vi "Device Level, Process Single Pulse.vi"(5 "filepath":path, 6 "Waveform Filtered Zoom":bool=TRUE, 7 "Waveform Zoom":bool, 8 "error in":errorcluster, 9 "Average Size":dbl=15.0, 10 "Resistance (ohms)":dbl=500.0 format="%.1f", 11 "waveform array":waveform(dbl)={"t0"=timestamp(3474563448.844 s since 1904-01-01), "dt"=4e-06, "Y"=[]}) -> (0 "error out":errorcluster, 1 "Input Parameters":T1[](array[typedef]) {"Value" format="%#.3f"}, 2 "Results":T1[](array[typedef]) {"Value" format="%#.3f"}, 3 "waveform filtered":waveform(dbl)(graph)={"t0"=timestamp(3472747248.0780005 s since 1904-01-01), "dt"=2e-06, "Y"=[]})   [LabVIEW 2010]
doc: "This function processes a single pulse waveform."
uses:
  Generic/Waveform Attribute/Waveform Attribute Cluster.ctl
panel:
  out "waveform":waveform(dbl)(graph)={"t0"=timestamp(3473168095.069 s since 1904-01-01), "dt"=2e-06, "Y"=[]}
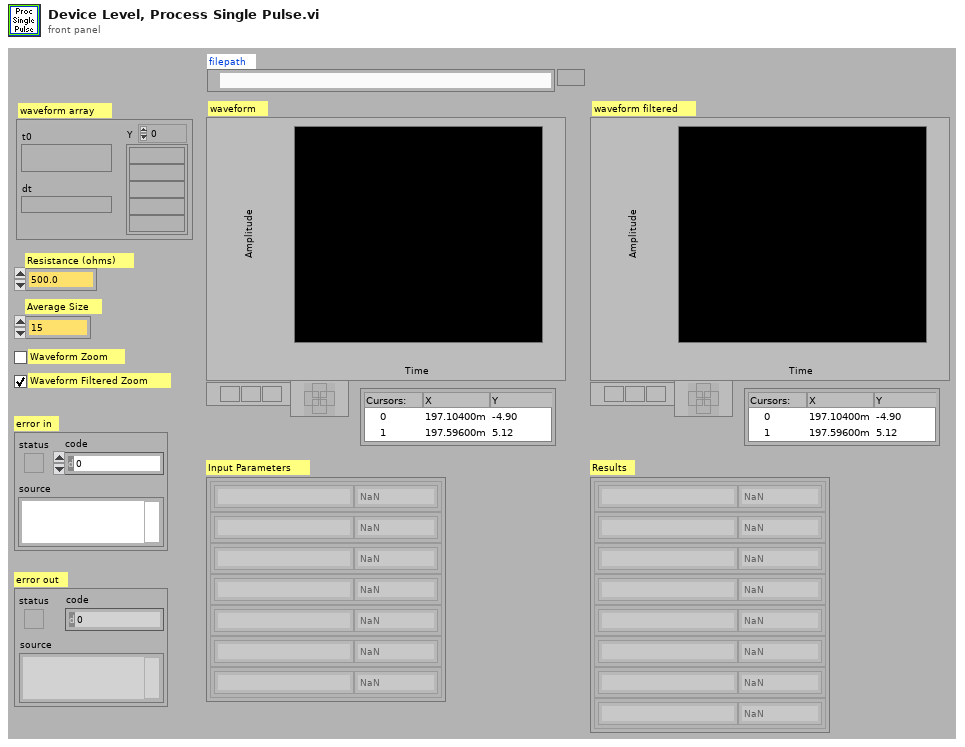
[diagram p1: front panel]
types:
  T1 = typedef "Waveform Attribute Cluster.ctl" = cluster{"Label":string, "Value":dbl}
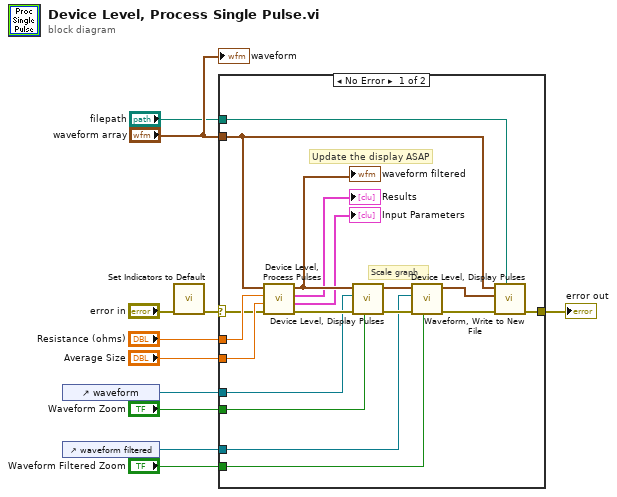
[diagram p0: block diagram]
diagram:
  n1 = control-ref of="waveform"() -> (w10:refnum<vi>)
  n2 = control-ref of="waveform filtered"() -> (w9:refnum<vi>)
  n3 = call "Set Indicators to Default.vi"("error in"="error in") -> ("error out"=w3:errorcluster)  [unwired: 6 in]
  n4 = case shown="No Error" w3 {
    selector: w3 -> [w17 w30]
    tunnel: [w15 w30] -> w11
    tunnel: w10 -> [w26 _]
    tunnel: w9 -> [w25 _]
    tunnel: "Waveform Zoom" -> [w24 _]
    tunnel: "Waveform Filtered Zoom" -> [w23 _]
    tunnel: "Resistance (ohms)" -> [w21 _]
    tunnel: "Average Size" -> [w20 _]
    tunnel: "waveform array" -> [w14 _]
    tunnel: "filepath" -> [w12 _]
    frame No Error {
      # "Update the display ASAP"
      # "Scale graph"
      n5 = call "Device Level, Process Pulses.vi"("error in"=w17, "Average Size"=w20, "Resistance (ohms)"=w21, "waveform"=w14) -> ("error out"=w29:errorcluster, "Input Parameters"=→"Input Parameters":T1[], "Results"=→"Results":T1[], "waveform out"=w22:waveform(dbl))  [unwired: 2 in]
      "waveform filtered" <- w22
      n6 = call "Device Level, Display Pulses.vi"("error in"=w29, "WFGraph Refnum"=w26, "waveform"=w22, "Zoom (F)"=w24) -> ("error out"=w28:errorcluster, "waveform dup"=w27:waveform(dbl))  [unwired: 5 in]
      n7 = call "Device Level, Display Pulses.vi"("error in"=w28, "WFGraph Refnum"=w25, "waveform"=w27, "Zoom (F)"=w23) -> ("error out"=w16:errorcluster, "waveform dup"=w13:waveform(dbl))  [unwired: 5 in]
      n8 = call "Waveform, Write to New File.vi"("filepath"=w12, "error in"=w16, "prc waveform"=w13, "raw waveform"=w14) -> ("error out"=w15:errorcluster)  [unwired: 2 in, 3 out]
    }
    frame Error {
    }
  }
  "error out" <- w11
  "waveform" <- "waveform array"
